vi "3_6.vi"() -> ()   [LabVIEW 2012]
panel:
  in  "Введення":bool[][](array[boolean])
  out "Генерація":bool[][](array[boolean])
  out "Результати":bool[][](array[boolean])
  in  "stop":bool
  in  "OK Button":bool
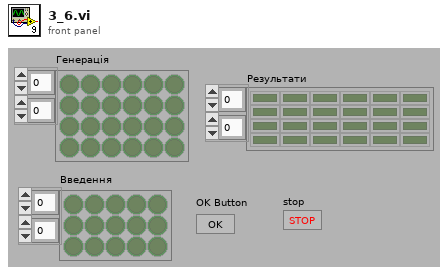
[diagram p1: front panel]
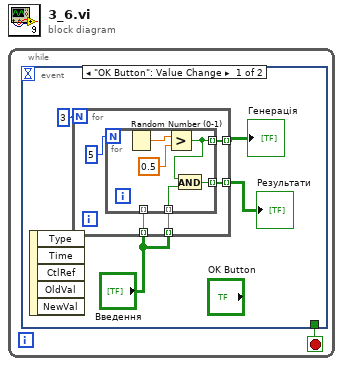
[diagram p0: block diagram]
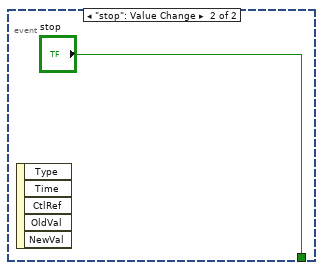
[diagram p2: hidden frame]
diagram:
  n1 = while {
    stop <- w1 stop-if-true
    n2 = event shown="[0] \"OK Button\": Value Change" {
      selector: _ -> [_ _]
      dyn-events: _ -> [_ _]
      timeout: _ -> [_ _]
      tunnel: [_ "stop"] -> w1
      event "OK Button": Value Change {
        n3 = event-data() -> ()  [unwired: 1 in, 5 out]
        n4 = for {
          N: 3 -> [_]
          tunnel: [w9] -> w4 mode=indexing
          tunnel: "Введення" -> [w8] mode=indexing
          tunnel: "Введення" -> [w7] mode=indexing
          tunnel: [w6] -> w2 mode=indexing
          n5 = for {
            N: 5 -> [_]
            tunnel: [w12] -> w9 mode=indexing
            tunnel: w8 -> [_] mode=indexing
            tunnel: w7 -> [w13] mode=indexing
            tunnel: [w11] -> w6 mode=indexing
            n6 = Random Number (0-1)() -> (number: 0 to 1=w15:dbl)
            n7 = Greater?(x=w15, y=0.5) -> (0:w12:bool)
            n8 = And(x=w12, y=w13) -> (x .and. y?=w11:bool)
          }
        }
        "Результати" <- w2
        "Генерація" <- w4
      }
      event "stop": Value Change {
        n9 = event-data() -> ()  [unwired: 1 in, 5 out]
      }
    }
  }
